vi "M13_Intake_Hardware.vi"   [LabVIEW 2019]
uses:
  Globals/Intake_Globals.vi
  Globals/Solenoid Globals.vi
  <vilib>/Rock Robotics/WPI/ThirdParty/REV Robotics/SPARK MAX/Typedef/Spark MAX Control Type.ctl
  <vilib>/Rock Robotics/WPI/Solenoid/WPI_SolenoidSetEnum.vi
types:
  T1 = typedef "WPI_MotorControlDeviceRef.ctl" = cluster{"DeviceStatus":errorcluster, "Type":T2, "PWM":cluster{"PWM Channel":T3, "DeadBand":T4}, "CAN":cluster{"Device Number":u8, "SetOutput VI Ref":variant, "GetOutput VI Ref":variant, "Enable VI Ref":variant, "Disable VI Ref":variant, "Data":variant}, "Invert":bool, "DIO PWM":cluster{"PWM \"Enable\" Channel":T3, "DIOChannel":T5, "PWM Rate":dbl}}
  T2 = typedef "WPI_MotorControlType.ctl" = enum16{"PWM", "CAN", "DIO PWM"}
  T3 = typedef "FPGA_DIOPWMChannel.ctl" = enum8{"PWM 0", "PWM 1", "PWM 2", "PWM 3", "PWM 4", "PWM 5", "PWM 6", "PWM 7", "PWM 8", "PWM 9", "PWM MXP 0", "PWM MXP 1", "PWM MXP 2", "PWM MXP 3", "PWM MXP 4", "PWM MXP 5", "PWM MXP 6", "PWM MXP 7", "PWM MXP 8", "PWM MXP 9", "Invalid"}
  T4 = typedef "WPI_PWMDeadband.ctl" = cluster{"Name":string, "maxPositivePwm":i32, "minPositivePwm":i32, "centerPwm":i32, "maxNegativePwm":i32, "minNegativePwm":i32, "angularRange":u16}
  T5 = typedef "FPGA_DIOChannel.ctl" = enum8{"DIO 0", "DIO 1", "DIO 2", "DIO 3", "DIO 4", "DIO 5", "DIO 6", "DIO 7", "DIO 8", "DIO 9", "DIO MXP 0", "DIO MXP 1", "DIO MXP 2", "DIO MXP 3", "DIO MXP 4", "DIO MXP 5", "DIO MXP 6", "DIO MXP 7", "DIO MXP 8", "DIO MXP 9", "DIO MXP 10", "DIO MXP 11", "DIO MXP 12", "DIO MXP 13", "DIO MXP 14", "DIO MXP 15", "SPI Port CS1", "SPI Port CS2", "SPI Port CS3", "SPI Port MISO", "SPI Port MOSI", "Invalid"}
  T6 = typedef "WPI_SolenoidDevRef.ctl" = cluster{"DevStatus":errorcluster, "Pneumatics Control Module":u8, "Forward Solenoid Channel":T7, "Reverse Solenoid Channel":T7}
  T7 = typedef "WPI_SolenoidChannel.ctl" = enum8{"Solenoid 0", "Solenoid 1", "Solenoid 2", "Solenoid 3", "Solenoid 4", "Solenoid 5", "Solenoid 6", "Solenoid 7", "Invalid"}
  T8 = typedef "Spark MAX Control Type.ctl" = enum16{"Percent VBus", "Voltage", "Velocity", "Position", "Smart Motion", "Current", "Smart Velocity"}
  T9 = typedef "Basic_Motor_Modes.ctl" = enum16{"Percent_Voltage", "Speed_Control", "Position_Control", "Current"}
  T10 = typedef "WPI_SolenoidValue.ctl" = enum16{"Off", "On", "Forward", "Reverse"}
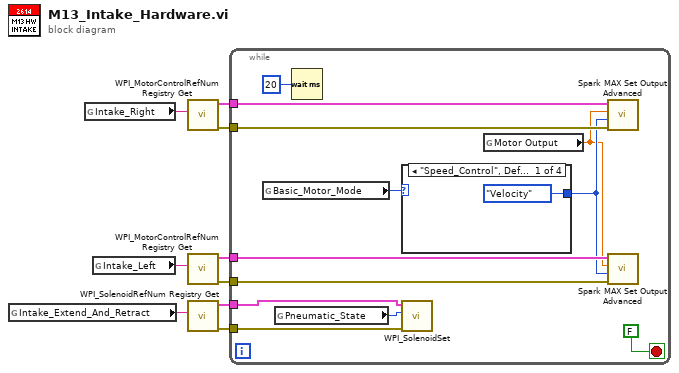
[diagram p0: block diagram]
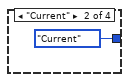
[diagram p2: hidden frame]
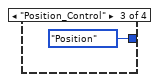
[diagram p3: hidden frame]
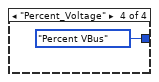
[diagram p4: hidden frame]
diagram:
  n1 = global read "Solenoid Globals.vi" "Intake_Extend_And_Retract"() -> (w9:string)
  n2 = global read "Intake_Globals.vi" "Intake_Right"() -> (w8:string)
  n3 = global read "Intake_Globals.vi" "Intake_Left"() -> (w7:string)
  n4 = call <vilib>:"WPI_MotorControlRefNum Registry Get.vi"("refnum name"=w8) -> ("error out"=w3:errorcluster, "MotorControlDevRef"=w5:T1)  [unwired: 9 in]
  n5 = call <vilib>:"WPI_MotorControlRefNum Registry Get.vi"("refnum name"=w7) -> ("error out"=w4:errorcluster, "MotorControlDevRef"=w6:T1)  [unwired: 9 in]
  n6 = call <vilib>:"WPI_SolenoidRefNum Registry Get.vi"("refnum name"=w9) -> ("error out"=w1:errorcluster, "SolenoidDevRef"=w2:T6)  [unwired: 9 in]
  n7 = while {
    tunnel: w6 -> [w18]
    tunnel: w5 -> [w17]
    tunnel: w4 -> [w16]
    tunnel: w3 -> [w15]
    tunnel: w2 -> [w12]
    tunnel: w1 -> [w10]
    stop <- FALSE stop-if-true
    n8 = global read "Intake_Globals.vi" "Basic_Motor_Mode"() -> (w19:T9)
    n9 = global read "Intake_Globals.vi" "Pneumatic_State"() -> (w11:T10)
    n10 = Wait (ms)(milliseconds to wait=u32 20) -> ()  [unwired: 1 out]
    n11 = case shown="\"Speed_Control\", Default" w19 {
      tunnel: [Spark_MAX_Control_Type."Velocity" ("Control Mode") Spark_MAX_Control_Type."Current" ("Control Mode") Spark_MAX_Control_Type."Position" ("Control Mode") Spark_MAX_Control_Type."Percent VBus" ("Control Mode")] -> w14
      frame "Speed_Control", Default {
      }
      frame "Current" {
      }
      frame "Position_Control" {
      }
      frame "Percent_Voltage" {
      }
    }
    n12 = call-poly <vilib>:"WPI_SolenoidSet.vi"("error in (no error)"=w10, "Value"=w11, "SolenoidDevRef"=w12) -> ()  [unwired: 7 in, 2 out]
    n13 = global read "Intake_Globals.vi" "Motor Output"() -> (w13:dbl)
    n14 = call <vilib>:"Spark MAX Set Output Advanced.vi"("error in (no error)"=w15, "Control Mode"=w14, "Setpoint"=w13, "MotorControlDevRef"=w17) -> ()  [unwired: 6 in, 2 out]
    n15 = call <vilib>:"Spark MAX Set Output Advanced.vi"("error in (no error)"=w16, "Control Mode"=w14, "Setpoint"=w13, "MotorControlDevRef"=w18) -> ()  [unwired: 6 in, 2 out]
  }
